vi "test.vi"   [LabVIEW 2017]
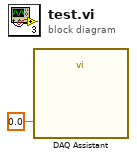
[diagram p0: block diagram]
diagram:
  n1 = call "DAQ Assistant"("data"=0.0) -> ()  [unwired: 17 in, 2 out]
